vi "MessageBase.getBytes.vi"(8 "error in (no error)":errorcluster, 11 "MessageBase in":refnum<class "MessageBase.lvclass">) -> (0 "error out":errorcluster, 2 "Bytes.out":u8[](array[numeric]), 3 "MessageBase out":refnum<class "MessageBase.lvclass">)   [LabVIEW 2022 SP3, in "MessageBase.lvclass"]
uses:
  MessageBase.lvclass
  FieldSpec.ctl
panel:
  out "reversed array":u8[](array[numeric])
  out "OrderedFieldSpecs":T1[](array[typedef])
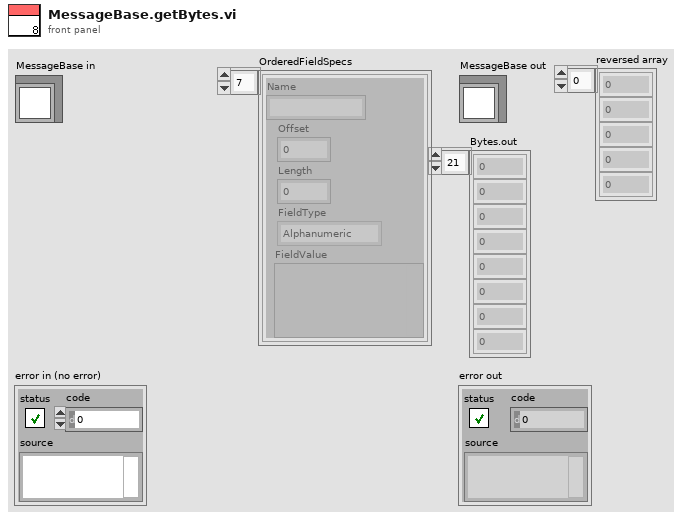
[diagram p1: front panel]
types:
  T1 = typedef "FieldSpec.ctl" = cluster{"Name":string, "Offset":i32, "Length":i32, "FieldType":enum16{"Alphanumeric", "Binary", "BinaryLongPrice", "BinaryShortPrice", "BitField", "PrintableAscii", "Value"}, "FieldValue":variant}
  T2 = enum16{"Alphanumeric", "Binary", "BinaryLongPrice", "BinaryShortPrice", "BitField", "PrintableAscii", "Value"}
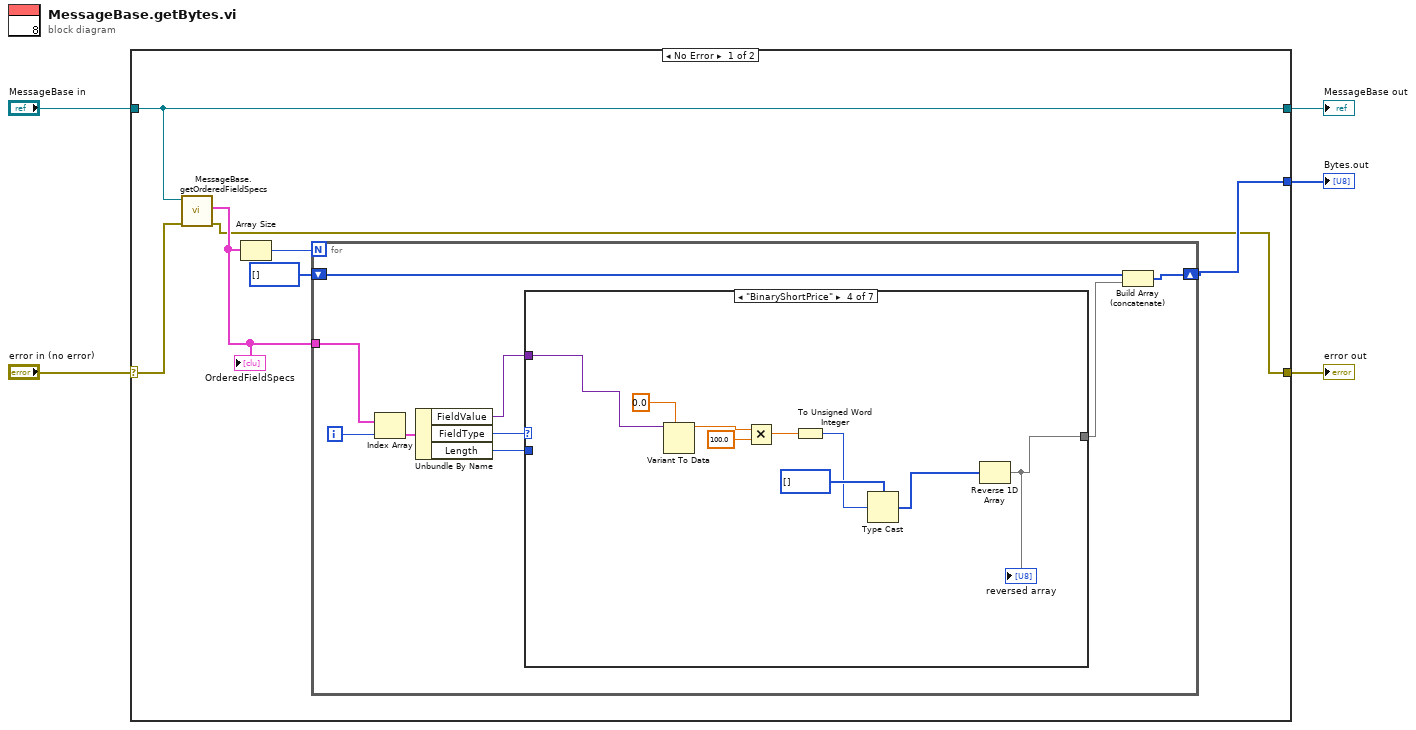
[diagram p0: block diagram]
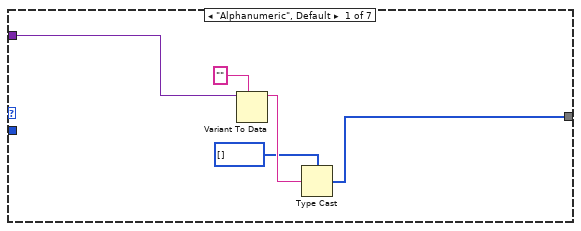
[diagram p2: hidden frame]
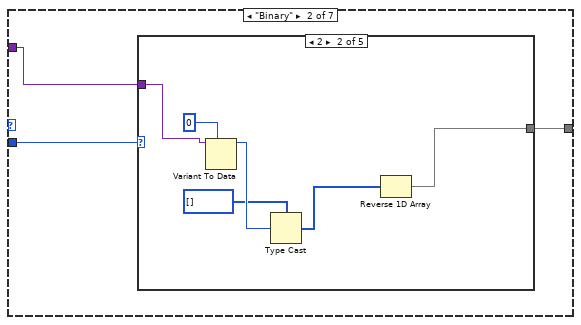
[diagram p3: hidden frame]
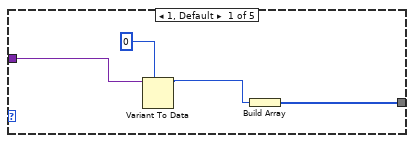
[diagram p4: hidden frame]
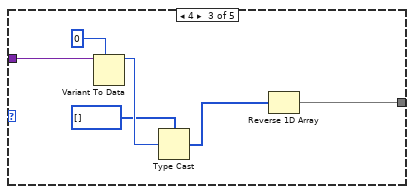
[diagram p5: hidden frame]
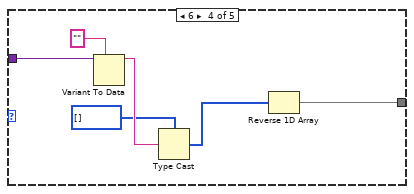
[diagram p6: hidden frame]
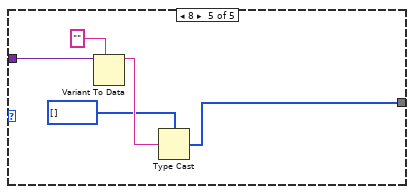
[diagram p7: hidden frame]
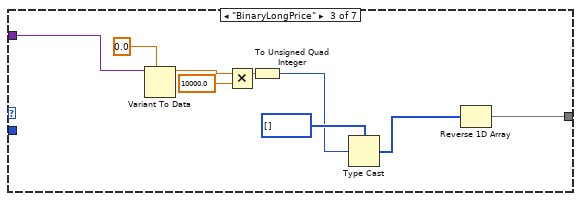
[diagram p8: hidden frame]
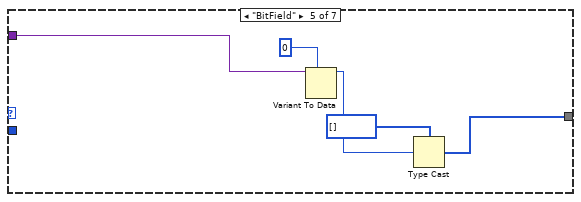
[diagram p9: hidden frame]
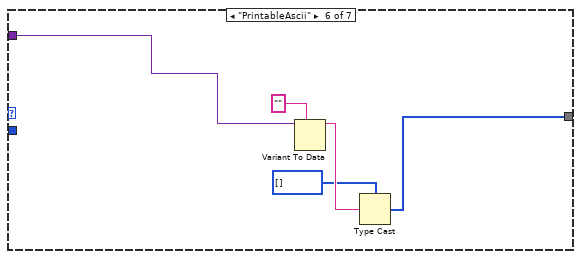
[diagram p10: hidden frame]
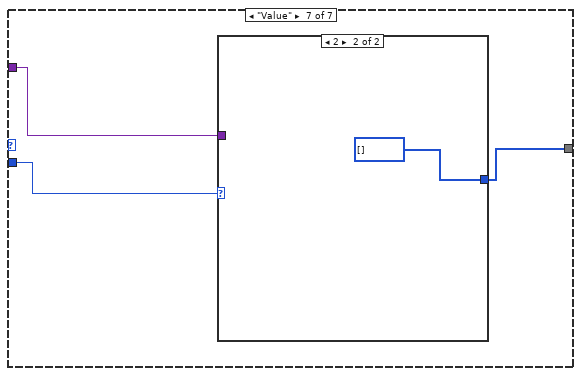
[diagram p11: hidden frame]
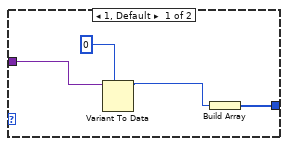
[diagram p12: hidden frame]
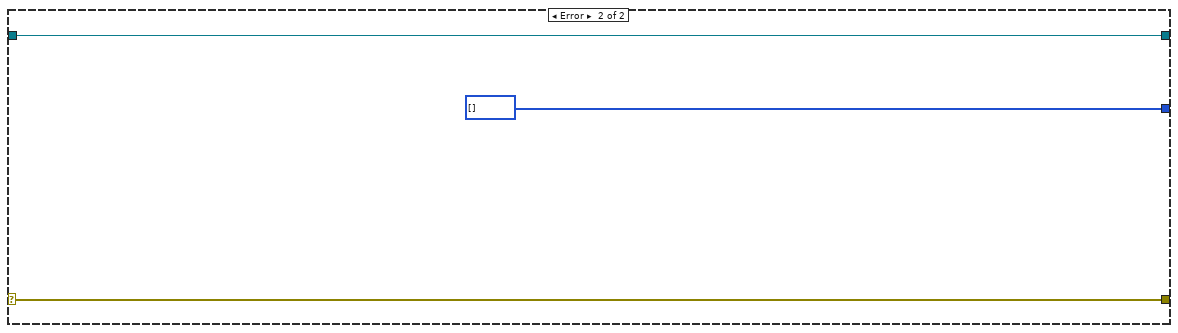
[diagram p13: hidden frame]
diagram:
  n1 = case shown="No Error" "error in (no error)" {
    selector: "error in (no error)" -> [w11 w95]
    tunnel: [w6 w95] -> w4
    tunnel: [w12 w94] -> w2
    tunnel: "MessageBase in" -> [w12 w94]
    tunnel: [w7 u8[] []] -> w1
    frame No Error {
      n2 = call-dynamic "MessageBase.getOrderedFieldSpecs.vi"("error in (no error)"=w11, "MessageBase in"=w12) -> ("error out"=w6:errorcluster, "OrderedFieldSpecs"=w8:T1[])  [unwired: 7 in, 1 out]
      "OrderedFieldSpecs" <- w8
      n3 = Array Size(array=w8) -> (size(s)=w9:i32)
      n4 = for {
        N: w9 -> [_]
        tunnel: w8 -> [w14]
        shift-right: [w17] -> w7
        shift-left: u8[] [] -> [w18]
        i -> [w15]
        n5 = Index Array(array=w14, index=w15) -> (element=w21:T1)
        n6 = Unbundle By Name(w21) -> ("FieldValue"=w13:variant, "FieldType"=w20:T2, "Length"=w19:i32)
        n7 = case shown="\"BinaryShortPrice\"" w20 {
          tunnel: w19 -> [_ w29 _ _ _ _ w86]
          tunnel: w13 -> [w23 w28 w62 w66 w76 w80 w87]
          tunnel: [w22 w27 w60 w67 w77 w81 w85] -> w16
          frame "Alphanumeric", Default {
            n8 = Variant To Data(type="", Variant=w23) -> (data=w25:string)  [unwired: 1 in, 1 out]
            n9 = Type Cast(type=u8[] [], x=w25) -> (*(type *) &x=w22:u8[])
          }
          frame "Binary" {
            n10 = case shown="2" w29 {
              tunnel: w28 -> [w33 w34 w44 w50 w55]
              tunnel: [w30 w35 w40 w46 w52] -> w27
              frame 1, Default {
                n11 = Variant To Data(type=u8 0, Variant=w33) -> (data=w31:u8)  [unwired: 1 in, 1 out]
                n12 = Build Array(w31) -> (w30:u8[])
              }
              frame 2 {
                n13 = Variant To Data(type=u16 0, Variant=w34) -> (data=w38:u16)  [unwired: 1 in, 1 out]
                n14 = Type Cast(type=u8[] [], x=w38) -> (*(type *) &x=w36:u8[])
                n15 = Reverse 1D Array(array=w36) -> (reversed array=w35:u8[])
              }
              frame 4 {
                n16 = Variant To Data(type=u32 0, Variant=w44) -> (data=w43:u32)  [unwired: 1 in, 1 out]
                n17 = Type Cast(type=u8[] [], x=w43) -> (*(type *) &x=w41:u8[])
                n18 = Reverse 1D Array(array=w41) -> (reversed array=w40:u8[])
              }
              frame 6 {
                n19 = Variant To Data(type="", Variant=w50) -> (data=w49:string)  [unwired: 1 in, 1 out]
                n20 = Type Cast(type=u8[] [], x=w49) -> (*(type *) &x=w47:u8[])
                n21 = Reverse 1D Array(array=w47) -> (reversed array=w46:u8[])
              }
              frame 8 {
                n22 = Variant To Data(type="", Variant=w55) -> (data=w54:string)  [unwired: 1 in, 1 out]
                n23 = Type Cast(type=u8[] [], x=w54) -> (*(type *) &x=w52:u8[])
              }
            }
          }
          frame "BinaryLongPrice" {
            n24 = Variant To Data(type=0.0, Variant=w62) -> (data=w65:dbl)  [unwired: 1 in, 1 out]
            n25 = Multiply(x=w65, y=10000.0) -> (x*y=w58:dbl)
            n26 = To Unsigned Quad Integer(1:w58) -> (0:w59:u64)
            n27 = Type Cast(type=u8[] [], x=w59) -> (*(type *) &x=w61:u8[])
            n28 = Reverse 1D Array(array=w61) -> (reversed array=w60:u8[])
          }
          frame "BinaryShortPrice" {
            n29 = Variant To Data(type=0.0, Variant=w66) -> (data=w74:dbl)  [unwired: 1 in, 1 out]
            n30 = Multiply(x=w74, y=100.0) -> (x*y=w69:dbl)
            n31 = To Unsigned Word Integer(number=w69) -> (unsigned 16bit integer=w70:u16)
            n32 = Type Cast(type=u8[] [], x=w70) -> (*(type *) &x=w71:u8[])
            n33 = Reverse 1D Array(array=w71) -> (reversed array=w67:u8[])
            "reversed array" <- w67
          }
          frame "BitField" {
            n34 = Variant To Data(type=u8 0, Variant=w76) -> (data=w75:u8)  [unwired: 1 in, 1 out]
            n35 = Type Cast(type=u8[] [], x=w75) -> (*(type *) &x=w77:u8[])
          }
          frame "PrintableAscii" {
            n36 = Variant To Data(type="", Variant=w80) -> (data=w83:string)  [unwired: 1 in, 1 out]
            n37 = Type Cast(type=u8[] [], x=w83) -> (*(type *) &x=w81:u8[])
          }
          frame "Value" {
            n38 = case shown="2" w86 {
              tunnel: w87 -> [w91 _]
              tunnel: [w88 u8[] []] -> w85
              frame 1, Default {
                n39 = Variant To Data(type=u8 0, Variant=w91) -> (data=w89:u8)  [unwired: 1 in, 1 out]
                n40 = Build Array(w89) -> (w88:u8[])
              }
              frame 2 {
              }
            }
          }
        }
        n41 = Build Array (concatenate)(w18, w16) -> (w17:u8[])
      }
    }
    frame Error {
    }
  }
  "error out" <- w4
  "MessageBase out" <- w2
  "Bytes.out" <- w1
